vi "merge_time_intervals.vi"(8 "error in (no error)":errorcluster, 10 "merging window size":dbl[unit], 11 "ImageCollection in":refnum<class "ImageCollection.lvclass">) -> (0 "error out":errorcluster, 3 "ImageCollection out":refnum<class "ImageCollection.lvclass">)   [LabVIEW 2010, in "ImageCollection.lvclass"]
uses:
  ImageCollection.lvclass
  Image/Image/Image.lvclass
  add_mode_enum.ctl
  ImageCollection.lvclass/ImageCollection.ctl
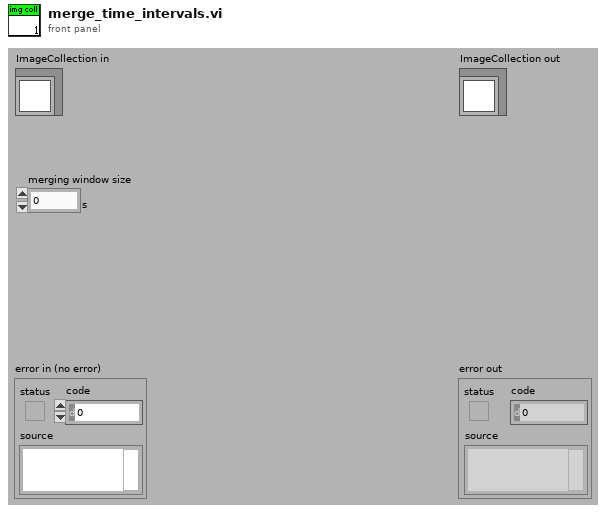
[diagram p1: front panel]
types:
  T1 = typedef "ImageCollection.lvclass/add_mode_enum.ctl" = enum16{"instance", "copy"}
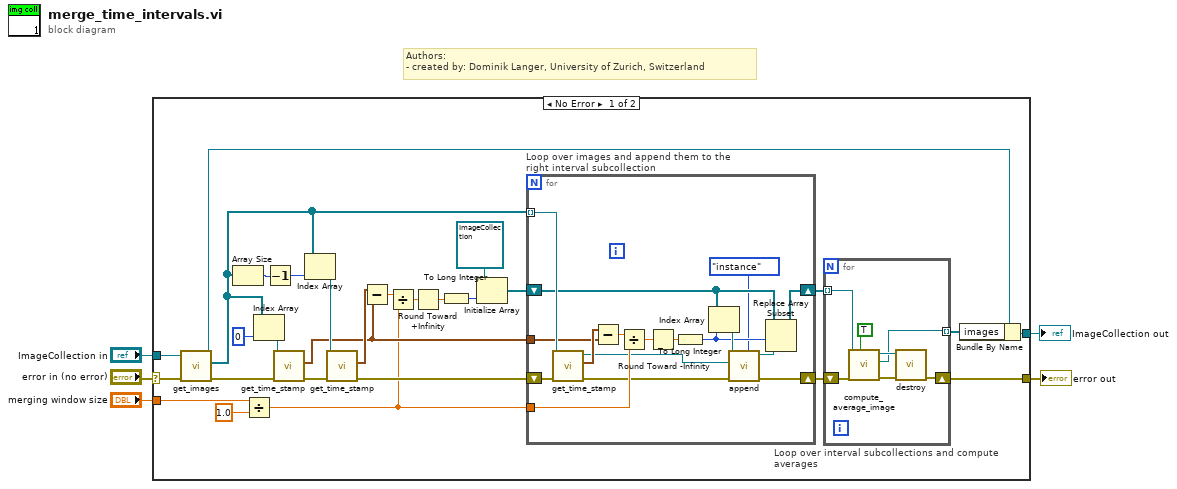
[diagram p0: block diagram]
diagram:
  # "Authors: \n- created by: Dominik Langer, University of Zurich, Switzerland"
  n1 = case shown="No Error" "error in (no error)" {
    selector: "error in (no error)" -> [w33 w59]
    tunnel: [w11 w59] -> w4
    tunnel: [w8 w58] -> w2
    tunnel: "ImageCollection in" -> [w32 w58]
    tunnel: "merging window size" -> [w31 _]
    frame No Error {
      n2 = call-dynamic "get_images.vi"("error in (no error)"=w33, "ImageCollection.lvclass in"=w32) -> ("error out"=w28:errorcluster, "images"=w26:refnum<class "Image.lvclass">[], "ImageCollection.lvclass out"=w9:refnum<class "ImageCollection.lvclass">)  [unwired: 7 out]
      n3 = Array Size(array=w26) -> (size(s)=w6:i32)
      n4 = Divide(x=w31, y=dbl[unit] 1.0) -> (x/y=w17:dbl)
      n5 = Index Array(array=w26, index=0) -> (element=w27:refnum<class "Image.lvclass">)
      n6 = Decrement(x=w6) -> (x-1=w7:i32)
      n7 = call-dynamic "get_time_stamp.vi"("error in (no error)"=w28, "Image.lvclass in"=w27) -> ("error out"=w25:errorcluster, "timestamp"=w18:timestamp)  [unwired: 8 out]
      n8 = Index Array(array=w26, index=w7) -> (element=w23:refnum<class "Image.lvclass">)
      n9 = call-dynamic "get_time_stamp.vi"("error in (no error)"=w25, "Image.lvclass in"=w23) -> ("error out"=w24:errorcluster, "timestamp"=w22:timestamp)  [unwired: 8 out]
      n10 = Subtract(x=w22, y=w18) -> (x-y=w21:dbl)
      n11 = Divide(x=w21, y=w17) -> (x/y=w16:dbl)
      n12 = Round Toward +Infinity(x=w16) -> (ceil(x): smallest int >= x=w15:dbl)
      n13 = To Long Integer(number=w15) -> (32bit integer=w20:i32)
      n14 = Initialize Array(refnum<class "ImageCollection.lvclass"> refnum ("ImageCollection.lvclass"), w20) -> (w19:refnum<class "ImageCollection.lvclass">[])
      n15 = for "Loop over images and append them to the right interval subcollection" {
        shift-right: [w42] -> w13
        shift-left: w24 -> [w57]
        tunnel: w26 -> [w56] mode=indexing
        shift-right: [w43] -> w12
        shift-left: w19 -> [w45]
        tunnel: w18 -> [w54]
        tunnel: w17 -> [w53]
        n16 = call-dynamic "get_time_stamp.vi"("error in (no error)"=w57, "Image.lvclass in"=w56) -> ("error out"=w49:errorcluster, "timestamp"=w55:timestamp, "Image.lvclass out"=w48:refnum<class "Image.lvclass">)  [unwired: 7 out]
        n17 = Subtract(x=w55, y=w54) -> (x-y=w52:dbl)
        n18 = Divide(x=w52, y=w53) -> (x/y=w51:dbl)
        n19 = Round Toward -Infinity(1:w51) -> (0:w50:dbl)
        n20 = To Long Integer(number=w50) -> (32bit integer=w44:i32)
        n21 = Index Array(array=w45, index=w44) -> (element=w46:refnum<class "ImageCollection.lvclass">)
        n22 = call-dynamic "append.vi"("add mode"=add_mode_enum."instance", "error in (no error)"=w49, "Image.lvclass"=w48, "ImageCollection in"=w46) -> ("error out"=w42:errorcluster, "ImageCollection out"=w47:refnum<class "ImageCollection.lvclass">)  [unwired: 6 out]
        n23 = Replace Array Subset(array=w45, new element=w47, index=w44) -> (w43:refnum<class "ImageCollection.lvclass">[])
      }
      n24 = for "Loop over interval subcollections and compute averages" {
        shift-right: [w34] -> w11
        shift-left: w13 -> [w40]
        tunnel: w12 -> [w37] mode=indexing
        tunnel: [w35] -> w10 mode=indexing
        n25 = call-dynamic "compute_average_image.vi"("all?"=TRUE, "error in (no error)"=w40, "ImageCollection in"=w37) -> ("error out"=w39:errorcluster, "averaged image"=w35:refnum<class "Image.lvclass">, "ImageCollection out"=w38:refnum<class "ImageCollection.lvclass">)  [unwired: 2 in, 4 out]
        n26 = call-dynamic "destroy.vi"("error in (no error)"=w39, "ImageCollection in"=w38) -> ("error out"=w34:errorcluster)  [unwired: 9 out]
      }
      n27 = Bundle By Name(cluster=w9, "images"=w10) -> (w8:refnum<class "ImageCollection.lvclass">)
    }
    frame Error {
    }
  }
  "error out" <- w4
  "ImageCollection out" <- w2
